vi "test Snapshot Operations.vi"(8 "error in (no error)":errorcluster, 11 "TestCase in":refnum<class "Test_Blob.lvclass">) -> (0 "error out":errorcluster, 3 "TestCase out":refnum<class "Test_Blob.lvclass">)   [LabVIEW 2015, in "Test_Blob.lvclass"]
uses:
  Test_Blob.lvclass
  Blob Storage/Blob Type.ctl
  Core/Name Value Pair.ctl
  Global Parameters.vi
  Core/Session/Session.lvclass
  Blob Storage/NI_Azure_Blob.lvlib
  Core/NI_Azure_Core.lvlib
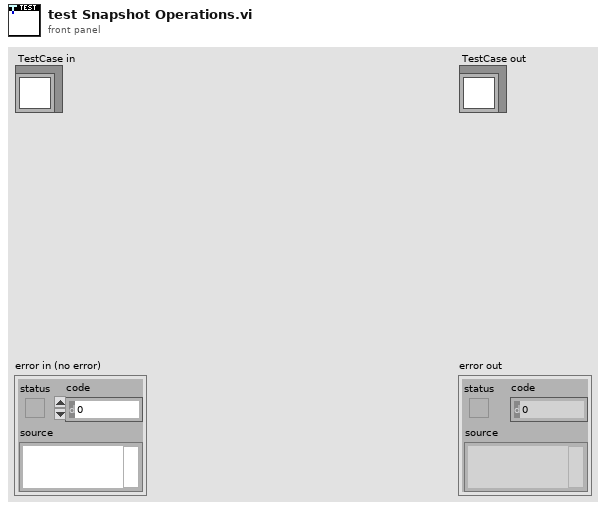
[diagram p1: front panel]
types:
  T1 = typedef "NI_Azure_Core.lvlib/Name Value Pair.ctl" = cluster{"name":string, "value":string}
  T2 = typedef "NI_Azure_Blob.lvlib/Blob Type.ctl" = enum16{"BlockBlob", "PageBlob", "AppendBlob"}
  T3 = typedef "NI_Azure_Core.lvlib/Azure Credentials.ctl" = cluster{"Storage Account Name":string, "Access Key":string}
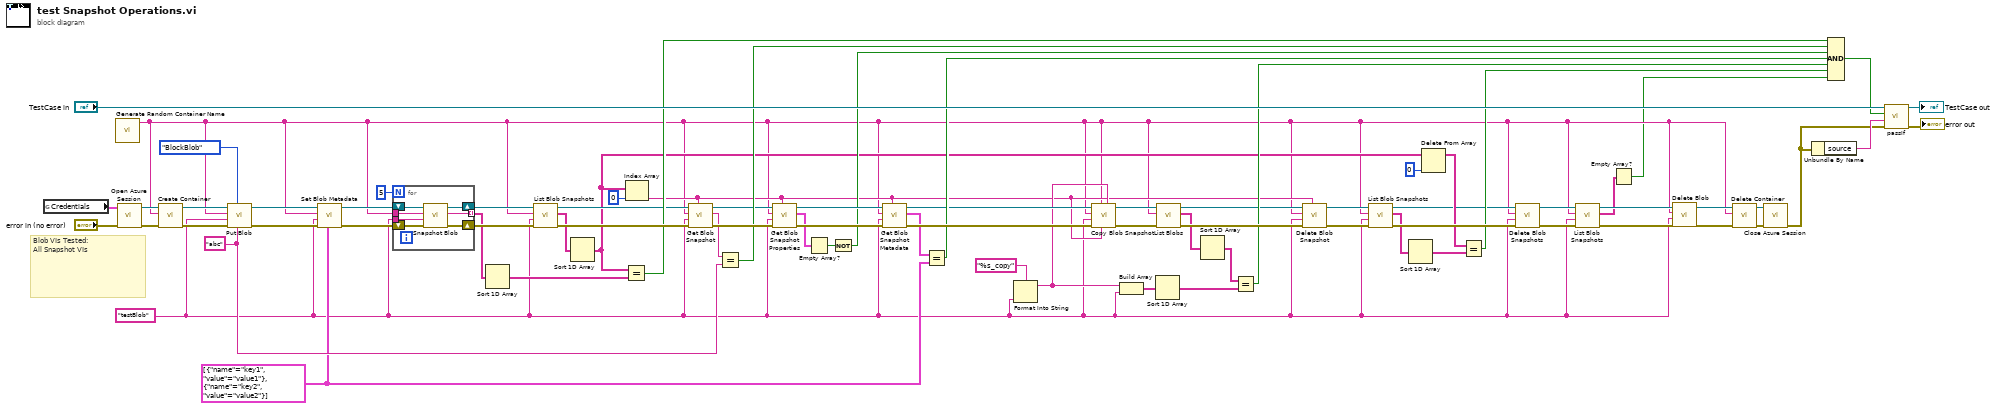
[diagram p0: block diagram]
diagram:
  w37 = T1[] [{"name"="key1", "value"="value1"}, {"name"="key2", "value"="value2"}] ("Blob Metadata")
  w44 = "abc" ("Block Content")
  w3 = "testBlob" ("Blob")
  # "Blob VIs Tested:\nAll Snapshot VIs"
  n1 = global read "Global Parameters.vi" "Credentials"() -> (w68:T3)
  n2 = call "Generate Random Container Name.vi"() -> ("Random Container Name"=w4:string)  [unwired: 11 in]
  n3 = call "Open Azure Session.vi"("error in (no error)"="error in (no error)", "Credentials"=w68) -> ("error out"=w69:errorcluster, "Azure Session"=w66:refnum<class "Session.lvclass">)  [unwired: 8 in]
  n4 = call "Create Container.vi"("error in (no error)"=w69, "Container"=w4, "Azure Session in"=w66) -> ("error out"=w72:errorcluster, "Azure Session out"=w71:refnum<class "Session.lvclass">)  [unwired: 7 in]
  n5 = call "Put Blob.vi"("Blob Content"=w44, "Blob type"=Blob_Type."BlockBlob", "error in (no error)"=w72, "Blob"=w3, "Container"=w4, "Azure Session in"=w71) -> ("error out"=w63:errorcluster, "Azure Session out"=w57:refnum<class "Session.lvclass">)  [unwired: 4 in]
  n6 = call "Set Blob Metadata.vi"("Blob Metadata"=w37, "error in (no error)"=w63, "Blob"=w3, "Container"=w4, "Azure Session in"=w57) -> ("error out"=w58:errorcluster, "Azure Session out"=w55:refnum<class "Session.lvclass">)  [unwired: 5 in]
  n7 = for {
    N: 5 -> [_]
    tunnel: w4 -> [w79]
    tunnel: w3 -> [w78]
    shift-right: [w82] -> w56
    shift-left: w58 -> [w83]
    shift-right: [w80] -> w52
    shift-left: w55 -> [w81]
    tunnel: [w77] -> w51 mode=indexing
    n8 = call "Snapshot Blob.vi"("error in (no error)"=w83, "Blob"=w78, "Container"=w79, "Azure Session in"=w81) -> ("error out"=w82:errorcluster, "Snapshot"=w77:string, "Azure Session out"=w80:refnum<class "Session.lvclass">)  [unwired: 5 in]
  }
  n9 = Sort 1D Array(array=w51) -> (sorted array=w49:string[])
  n10 = call "List Blob Snapshots.vi"("error in (no error)"=w56, "Blob name"=w3, "Container"=w4, "Azure Session in"=w52) -> ("error out"=w53:errorcluster, "Blob snapshots"=w50:string[], "Azure Session out"=w46:refnum<class "Session.lvclass">)  [unwired: 5 in]
  n11 = Sort 1D Array(array=w50) -> (sorted array=w16:string[])
  n12 = Equal?(x=w16, y=w49) -> (x = y?=w48:bool)
  n13 = Index Array(array=w16, index=0) -> (element=w19:string)
  n14 = call "Get Blob Snapshot.vi"("Snapshot"=w19, "error in (no error)"=w53, "Blob"=w3, "Container"=w4, "Azure Session in"=w46) -> ("error out"=w47:errorcluster, "Blob Content"=w45:string, "Azure Session out"=w41:refnum<class "Session.lvclass">)  [unwired: 4 in]
  n15 = Equal?(x=w45, y=w44) -> (x = y?=w43:bool)
  n16 = call "Get Blob Snapshot Properties.vi"("Snapshot"=w19, "error in (no error)"=w47, "Blob"=w3, "Container"=w4, "Azure Session in"=w41) -> ("error out"=w42:errorcluster, "Blob Properties"=w36:T1[], "Azure Session out"=w39:refnum<class "Session.lvclass">)  [unwired: 4 in]
  n17 = Empty Array?(array=w36) -> (empty?=w35:bool)
  n18 = Not(x=w35) -> (.not. x?=w34:bool)
  n19 = call "Get Blob Snapshot Metadata.vi"("Snapshot"=w19, "error in (no error)"=w42, "Blob"=w3, "Container"=w4, "Azure Session in"=w39) -> ("error out"=w40:errorcluster, "Blob Metadata"=w38:T1[], "Azure Session out"=w31:refnum<class "Session.lvclass">)  [unwired: 4 in]
  n20 = Equal?(x=w38, y=w37) -> (x = y?=w33:bool)
  n21 = Format Into String(format string="%s_copy", w3) -> (resulting string=w27:string)  [unwired: 2 in, 1 out]
  n22 = call "Copy Blob Snapshot.vi"("Destination Blob"=w27, "Snapshot"=w19, "Destination Container"=w4, "error in (no error)"=w40, "Source Blob"=w3, "Source Container"=w4, "Azure Session in"=w31) -> ("error out"=w32:errorcluster, "Azure Session out"=w28:refnum<class "Session.lvclass">)  [unwired: 2 in, 1 out]
  n23 = Build Array(w27, w3) -> (w26:string[])
  n24 = Sort 1D Array(array=w26) -> (sorted array=w23:string[])
  n25 = call "List Blobs.vi"("error in (no error)"=w32, "Container"=w4, "Azure Session in"=w28) -> ("error out"=w29:errorcluster, "Blobs"=w25:string[], "Azure Session out"=w20:refnum<class "Session.lvclass">)  [unwired: 6 in]
  n26 = Sort 1D Array(array=w25) -> (sorted array=w24:string[])
  n27 = Equal?(x=w24, y=w23) -> (x = y?=w22:bool)
  n28 = call "Delete Blob Snapshot.vi"("Snapshot"=w19, "error in (no error)"=w29, "Blob"=w3, "Container"=w4, "Azure Session in"=w20) -> ("error out"=w21:errorcluster, "Azure Session out"=w17:refnum<class "Session.lvclass">)  [unwired: 5 in]
  n29 = call "List Blob Snapshots.vi"("error in (no error)"=w21, "Blob name"=w3, "Container"=w4, "Azure Session in"=w17) -> ("error out"=w18:errorcluster, "Blob snapshots"=w13:string[], "Azure Session out"=w8:refnum<class "Session.lvclass">)  [unwired: 5 in]
  n30 = Sort 1D Array(array=w13) -> (sorted array=w11:string[])
  n31 = Delete From Array(array=w16, index=0) -> (array with subset deleted=w12:string[])  [unwired: 1 in, 1 out]
  n32 = Equal?(x=w12, y=w11) -> (x = y?=w10:bool)
  n33 = call "Delete Blob Snapshots.vi"("error in (no error)"=w18, "Blob"=w3, "Container"=w4, "Azure Session in"=w8) -> ("error out"=w9:errorcluster, "Azure Session out"=w6:refnum<class "Session.lvclass">)  [unwired: 6 in]
  n34 = call "List Blob Snapshots.vi"("error in (no error)"=w9, "Blob name"=w3, "Container"=w4, "Azure Session in"=w6) -> ("error out"=w7:errorcluster, "Blob snapshots"=w2:string[], "Azure Session out"=w5:refnum<class "Session.lvclass">)  [unwired: 5 in]
  n35 = Empty Array?(array=w2) -> (empty?=w1:bool)
  n36 = call "Delete Blob.vi"("error in (no error)"=w7, "Blob"=w3, "Container"=w4, "Azure Session in"=w5) -> ("error out"=w61:errorcluster, "Azure Session out"=w62:refnum<class "Session.lvclass">)  [unwired: 6 in]
  n37 = call "Delete Container.vi"("error in (no error)"=w61, "Container"=w4, "Azure Session in"=w62) -> ("error out"=w67:errorcluster, "Azure Session out"=w64:refnum<class "Session.lvclass">)  [unwired: 7 in]
  n38 = call "Close Azure Session.vi"("error in (no error)"=w67, "Azure Session"=w64) -> ("error out"=w65:errorcluster)  [unwired: 9 in]
  n39 = Unbundle By Name(w65) -> ("source"=w73:string)
  n40 = Compound Arithmetic op=AND(w48, w43, w34, w33, w22, w10, w1) -> (w60:bool)
  n41 = call-dynamic "passIf.vi"("error in (no error)"=w65, "message (\"\")"=w73, "pass"=w60, "TestCase in"="TestCase in") -> ("error out"=→"error out":errorcluster, "TestCase out"=→"TestCase out":refnum<class "Test_Blob.lvclass">)  [unwired: 6 in]
